vi "Weather Station Sandbox.vi"() -> ()   [LabVIEW 2011]
uses:
  Classes/Humidity Bricklet/Properties/Read CB humidity.vi
  Classes/Ambient Light Bricklet/Properties/Read CB illuminance.vi
  Classes/Temperature IR Bricklet/Properties/Read CB ambient temperature.vi
  Classes/Temperature IR Bricklet/Properties/Read CB object temperature.vi
  Classes/IP Connection/IP Connection.lvclass
  Classes/Ambient Light Bricklet/Ambient Light Bricklet.lvclass
  Classes/Humidity Bricklet/Humidity Bricklet.lvclass
  Classes/Temperature IR Bricklet/Temperature IR Bricklet.lvclass
panel:
  out "Illuminance":dbl format="%.1f Lux"
  out "Humidity":dbl format="%.1f %%"
  out "Object T.":dbl format="%.1f °C"
  out "Ambient T.":dbl format="%.1f °C"
  out "XY Graph":cluster{dbl[], dbl[]}[](graph)
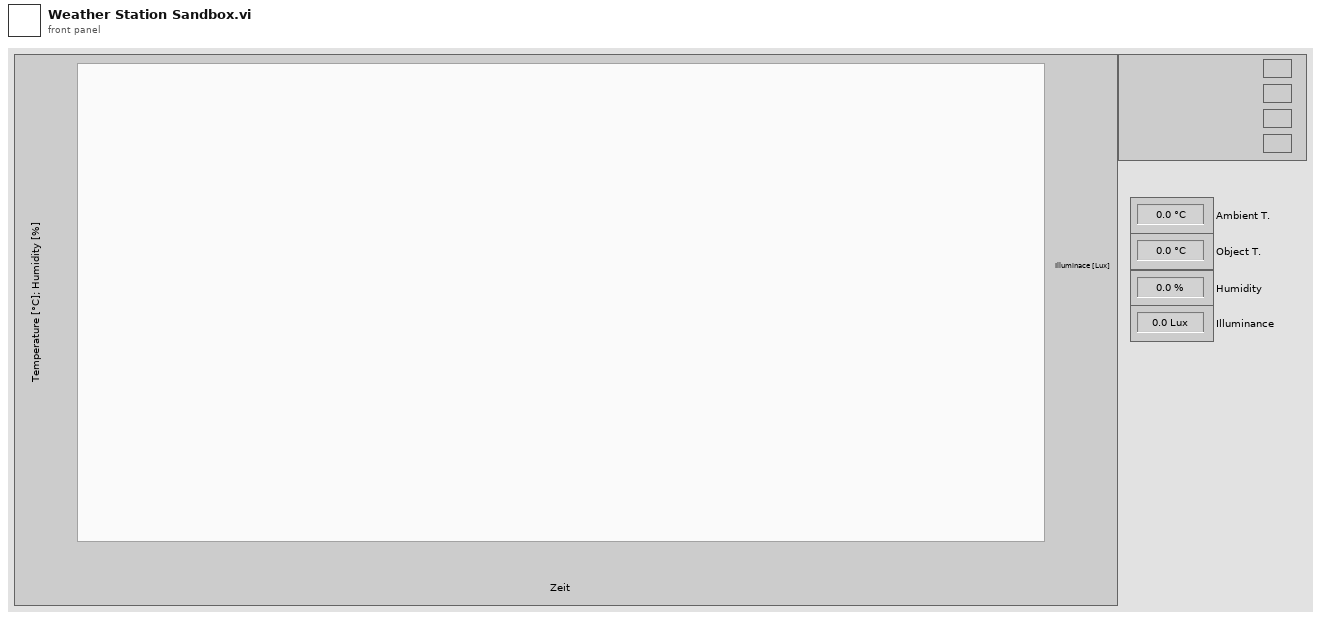
[diagram p1: front panel]
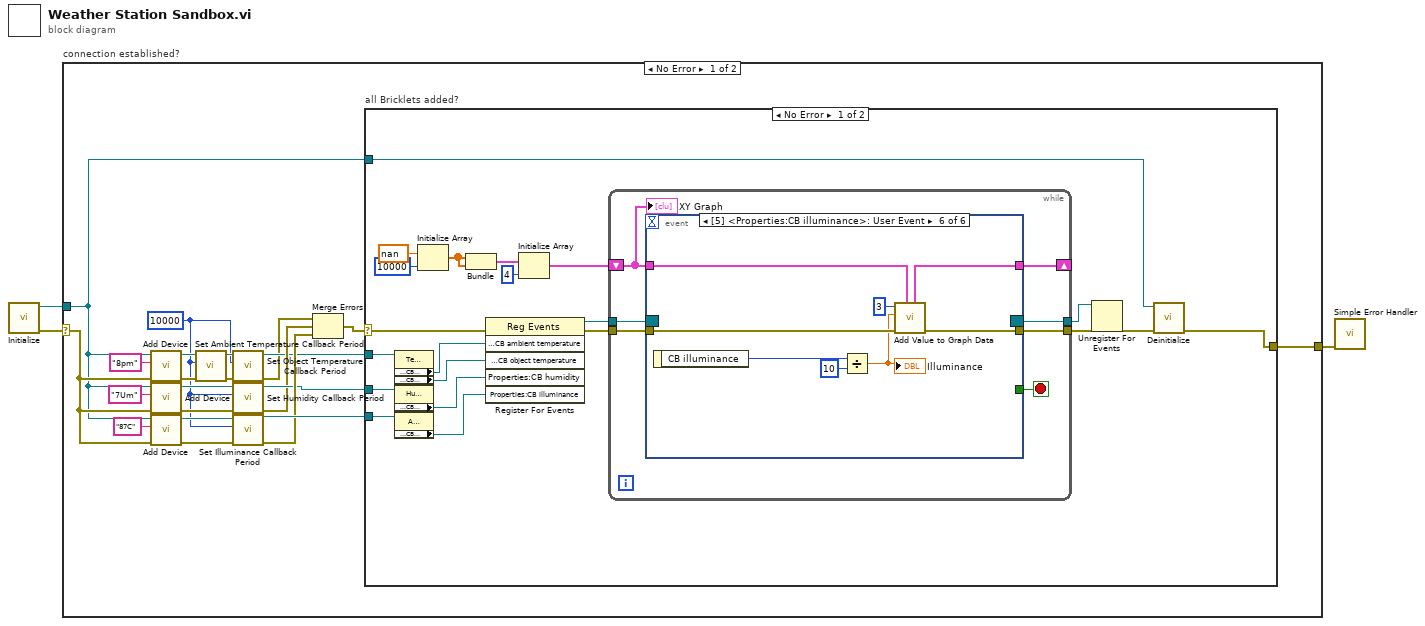
[diagram p0: block diagram]
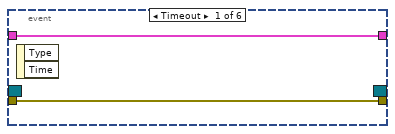
[diagram p2: hidden frame]
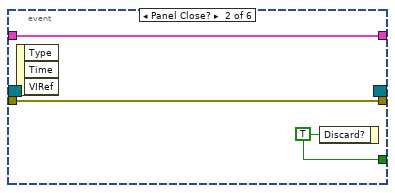
[diagram p3: hidden frame]
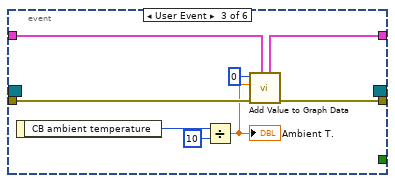
[diagram p4: hidden frame]
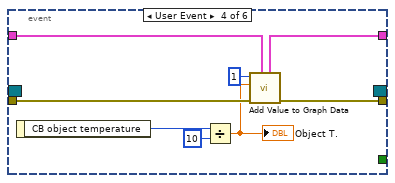
[diagram p5: hidden frame]
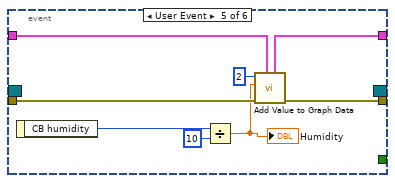
[diagram p6: hidden frame]
diagram:
  n1 = call "Initialize.vi"() -> ("error out"=w3:errorcluster, "IP Connection out"=w2:refnum<class "IP Connection.lvclass">)  [unwired: 10 in]
  n2 = case "connection established?" shown="No Error" w3 {
    selector: w3 -> [w22 w91]
    tunnel: w2 -> [w5 _]
    tunnel: [w6 w91] -> w1
    frame No Error {
      w7 = u32 10000 ("period (0: off)")
      n3 = call "Add Device.vi"("Error In"=w22, "Device UID"="8pm", "IP Connection"=w5) -> ("Error Out"=w12:errorcluster, "Ambient Light Bricklet"=w13:refnum<class "Temperature IR Bricklet.lvclass">)  [unwired: 7 in]
      n4 = call "Add Device.vi"("Error In"=w22, "Device UID"="7Um", "IP Connection"=w5) -> ("Error Out"=w17:errorcluster, "Humidity Bricklet"=w15:refnum<class "Humidity Bricklet.lvclass">)  [unwired: 7 in]
      n5 = call "Add Device.vi"("Error In"=w22, "Device UID"="87C", "IP Connection"=w5) -> ("Error Out"=w19:errorcluster, "Ambient Light Bricklet"=w21:refnum<class "Ambient Light Bricklet.lvclass">)  [unwired: 7 in]
      n6 = call "Set Ambient Temperature Callback Period.vi"("error in (no error)"=w12, "period (0: off)"=w7, "Temperature IR Bricklet in"=w13) -> ("error out"=w8:errorcluster, "Temperature IR Bricklet out"=w11:refnum<class "Temperature IR Bricklet.lvclass">)  [unwired: 7 in]
      n7 = call "Set Object Temperature Callback Period.vi"("error in (no error)"=w8, "period (0: off)"=w7, "Temperature IR Bricklet in"=w11) -> ("error out"=w9:errorcluster, "Temperature IR Bricklet out"=w10:refnum<class "Temperature IR Bricklet.lvclass">)  [unwired: 7 in]
      n8 = call "Set Humidity Callback Period.vi"("error in (no error)"=w17, "period (0: off)"=w7, "Humidity Bricklet in"=w15) -> ("error out"=w14:errorcluster, "Humidity Bricklet out"=w16:refnum<class "Humidity Bricklet.lvclass">)  [unwired: 7 in]
      n9 = call "Set Illuminance Callback Period.vi"("error in (no error)"=w19, "period (0: off)"=w7, "Ambient Light Bricklet in"=w21) -> ("error out"=w18:errorcluster, "Ambient Light Bricklet out"=w20:refnum<class "Ambient Light Bricklet.lvclass">)  [unwired: 7 in]
      n10 = Merge Errors(w9, w14, w18) -> (w4:errorcluster)
      n11 = case "all Bricklets added?" shown="No Error" w4 {
        selector: w4 -> [w33 w90]
        tunnel: w20 -> [w41 _]
        tunnel: w16 -> [w40 _]
        tunnel: w10 -> [w39 _]
        tunnel: [w26 w90] -> w6
        tunnel: w5 -> [w34 _]
        frame No Error {
          n12 = property class="Temperature IR Bricklet.lvclass"(reference=w39) -> ("Properties:CB ambient temperature"=w45:refnum<user-event>, "Properties:CB object temperature"=w44:refnum<user-event>)  [unwired: 1 in, 2 out]
          n13 = property class="Humidity Bricklet.lvclass"(reference=w40) -> ("Properties:CB humidity"=w43:refnum<user-event>)  [unwired: 1 in, 2 out]
          n14 = property class="Ambient Light Bricklet.lvclass"(reference=w41) -> ("Properties:CB illuminance"=w42:refnum<user-event>)  [unwired: 1 in, 2 out]
          n15 = Initialize Array(nan ("element"), 10000 ("dimension size")) -> (w30:dbl[])
          n16 = Bundle(w30, w30) -> (w29:cluster{dbl[], dbl[]})  [unwired: 1 in]
          n17 = register-events(error in=w33, w45, w44, w43, w42) -> (reference out=w37:refnum<event-registration>, error out=w38:errorcluster)  [unwired: 1 in]
          n18 = Initialize Array(w29, 4 ("dimension size")) -> (w27:cluster{dbl[], dbl[]}[])
          n19 = while {
            tunnel: w38 -> [w52]
            tunnel: w37 -> [w51]
            tunnel: [w50] -> w36
            tunnel: [w49] -> w35
            shift-right: [w46] -> _
            shift-left: w27 -> [w47]
            stop <- w48 stop-if-true
            n20 = event shown="[5] <Properties:CB illuminance>: User Event" {
              selector: w51 -> [_ _ _ _ _ _]
              dyn-events: [_ _ _ _ _ _] -> w50
              timeout: _ -> [_ _ _ _ _ _]
              tunnel: w52 -> [w54 w55 w63 w71 w79 w87]
              tunnel: [w54 w55 w62 w70 w78 w86] -> w49
              tunnel: [_ w57 _ _ _ _] -> w48
              tunnel: w47 -> [w53 w56 w61 w67 w75 w83]
              tunnel: [w53 w56 w60 w66 w74 w82] -> w46
              event Timeout {
                n21 = event-data() -> ()  [unwired: 1 in, 2 out]
              }
              event Panel Close? {
                w57 = TRUE ("Discard?")
                n22 = event-data() -> ()  [unwired: 1 in, 3 out]
                n23 = event-data("Discard?"=w57) -> ()  [unwired: 1 in, 1 out]
              }
              event User Event {
                n24 = event-data() -> ("CB ambient temperature"=w65:i16)  [unwired: 1 in]
                n25 = Divide(x=w65, y=i16 10) -> (x/y=w59:dbl)
                "Ambient T." <- w59
                n26 = call "Add Value to Graph Data.vi"("Graph Data in"=w61, "Error In"=w63, "Value"=w59, "Index"=0) -> ("Error Out"=w62:errorcluster, "Graph Data out"=w60:cluster{"Array":dbl[], "Array":dbl[]}[])  [unwired: 6 in]
              }
              event User Event {
                n27 = event-data() -> ("CB object temperature"=w73:i16)  [unwired: 1 in]
                n28 = Divide(x=w73, y=i16 10) -> (x/y=w69:dbl)
                "Object T." <- w69
                n29 = call "Add Value to Graph Data.vi"("Graph Data in"=w67, "Error In"=w71, "Value"=w69, "Index"=1) -> ("Error Out"=w70:errorcluster, "Graph Data out"=w66:cluster{"Array":dbl[], "Array":dbl[]}[])  [unwired: 6 in]
              }
              event User Event {
                n30 = event-data() -> ("CB humidity"=w81:u16)  [unwired: 1 in]
                n31 = Divide(x=w81, y=i16 10) -> (x/y=w77:dbl)
                "Humidity" <- w77
                n32 = call "Add Value to Graph Data.vi"("Graph Data in"=w75, "Error In"=w79, "Value"=w77, "Index"=2) -> ("Error Out"=w78:errorcluster, "Graph Data out"=w74:cluster{"Array":dbl[], "Array":dbl[]}[])  [unwired: 6 in]
              }
              event User Event {
                n33 = event-data() -> ("CB illuminance"=w89:u16)  [unwired: 1 in]
                n34 = Divide(x=w89, y=i16 10) -> (x/y=w85:dbl)
                "Illuminance" <- w85
                n35 = call "Add Value to Graph Data.vi"("Graph Data in"=w83, "Error In"=w87, "Value"=w85, "Index"=3) -> ("Error Out"=w86:errorcluster, "Graph Data out"=w82:cluster{"Array":dbl[], "Array":dbl[]}[])  [unwired: 6 in]
              }
            }
            "XY Graph" <- w47
          }
          n36 = Unregister For Events(event registration refnum=w36) -> ()  [unwired: 1 in, 1 out]
          n37 = call "Deinitialize.vi"("error in (no error)"=w35, "IP Connection in"=w34) -> ("error out"=w26:errorcluster)  [unwired: 9 in]
        }
        frame Error {
        }
      }
    }
    frame Error {
    }
  }
  n38 = call <vilib>:"Simple Error Handler.vi"("error in (no error)"=w1) -> ()  [unwired: 4 in, 5 out]
